vi "Decimate data.vi"(10 "Plot Area:Size:Width":i32=342, 11 "Plot (unix)":T1) -> (3 "Plot (unix)":T1)   [LabVIEW 2021, in "RocketPlot.lvlib"]
uses:
  RocketPlot.lvlib
  TypeDefs/plot datapoint.ctl
  10c546bb-84c8-4f1e-93dc-e9aef4c9908a.vi
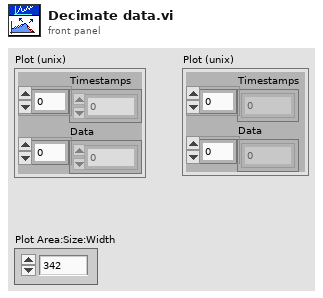
[diagram p1: front panel]
types:
  T1 = typedef "RocketPlot.lvlib/plot datapoint.ctl" = cluster{"Timestamps":u64[], "Data":dbl[]}
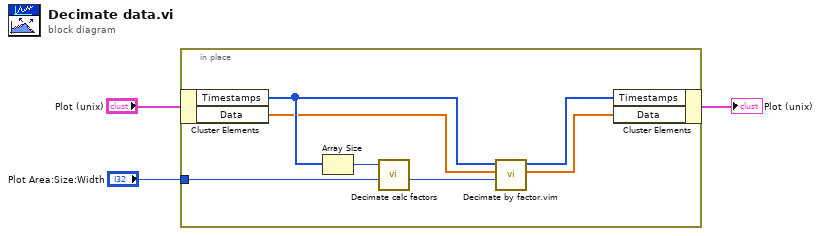
[diagram p0: block diagram]
diagram:
  n1 = in-place {
    in-place-border: "Plot Area:Size:Width" -> [w10]
    n2 = in-place-cluster #1("Plot (unix)") -> ("Timestamps"=w8:u64[], "Data"=w6:dbl[])
    n3 = Array Size(array=w8) -> (size(s)=w9:i32)
    n4 = call "Decimate calc factors.vi"("display width"=w10, "input buffer size"=w9) -> ("decimation factor"=w4:i32)  [unwired: 7 in, 2 out]
    n5 = call "Decimate by factor.vim"("decimation factor"=w4, "data Array"=w6, "time array"=w8) -> ("decimated data array"=w5:dbl[], "decimated time array"=w7:u64[])  [unwired: 6 in, 1 out]
    n6 = in-place-cluster #1("Timestamps"=w7, "Data"=w5) -> (→"Plot (unix)":T1)
  }
